vi "Config Measure Harmonics.vi"(0 "VISA resource name":refnum<visa-resource-name>, 5 "Harmonics Item (2: V)":u16(ring)=2 items=["Sync", "VTHD", "V", "VCON", "ATHD", "A", "ACON", "PF", "W", "WCON", "Vdeg", "Adeg"], 7 "State (F: OFF)":bool, 11 "error in (no error)":errorcluster) -> (4 "VISA resource name out":refnum<visa-resource-name>, 15 "error out":errorcluster)   [LabVIEW 2010, in "Yokogawa WT200 Series.lvlib"]
doc: "This VI sends the Harmonics Measurement command to the WT200 Series.\n\nNote : It needs /HRM option."
uses:
  G:/Engineering/Retail/LabV/instr.lib/Yokogawa WT200 Series/Yokogawa WT200 Series.lvlib
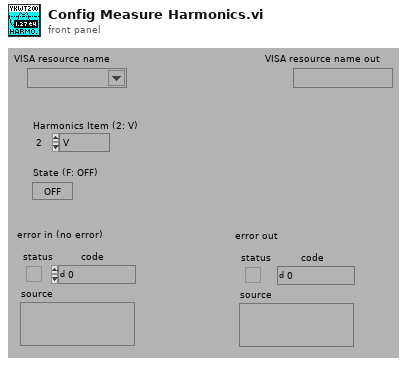
[diagram p1: front panel]
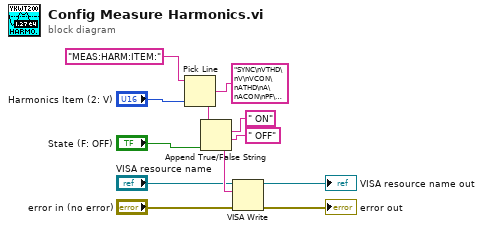
[diagram p0: block diagram]
diagram:
  n1 = Pick Line(string ("")="MEAS:HARM:ITEM:", multi-line string="SYNC\nVTHD\nV\nVCON\nATHD\nA\nACON\nPF\nW\nWCON\nVDEG\nADEG", line index="Harmonics Item (2: V)") -> (output string=w3:string)
  n2 = Append True/False String(1:"State (F: OFF)", 2:" OFF", 3:" ON", 4:w3) -> (0:w8:string)
  n3 = VISA Write(VISA resource name="VISA resource name", write buffer=w8, error in (no error)="error in (no error)") -> (VISA resource name out=→"VISA resource name out":refnum<visa-resource-name>, error out=→"error out":errorcluster)  [unwired: 1 out]
